vi "AddNewToneParamWave.vi"(1 "Phase  [°]":dbl format="%#_16g", 2 "Phase Selection":u16(ring) items=["Value", "Default", "Minimum", "Maximum"], 4 "Amplitude  [V]":dbl=1.0 format="%#_16g", 5 "Frequency [Hz]":dbl=1000000.0 format="%#_16e", 6 "Amplitude Selection":u16(ring) items=["Value", "Default", "Minimum", "Maximum"], 7 "Frequency Selection":u16(ring) items=["Value", "Default", "Minimum", "Maximum"], 8 "error in (no error)":errorcluster, 10 "ParamWave Name":string, 11 "VISA resource name":refnum<visa-resource-name>) -> (0 "error out":errorcluster, 3 "VISA resource name out":refnum<visa-resource-name>)   [LabVIEW 2020, in "Active Technologies AWG3000.lvlib"]
uses:
  Active Technologies AWG3000.lvlib
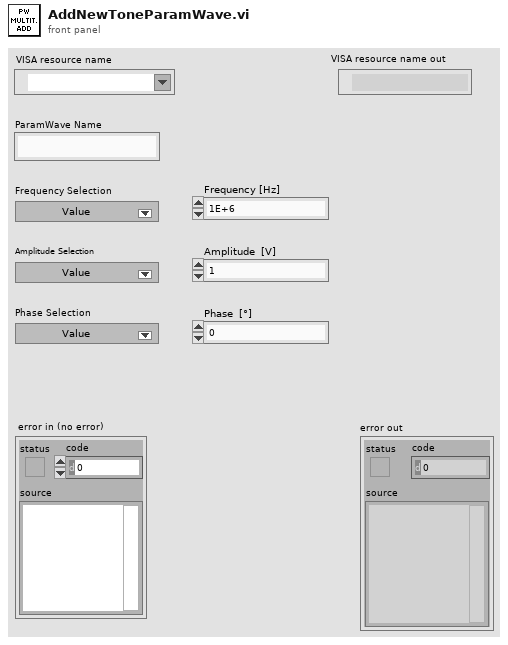
[diagram p1: front panel]
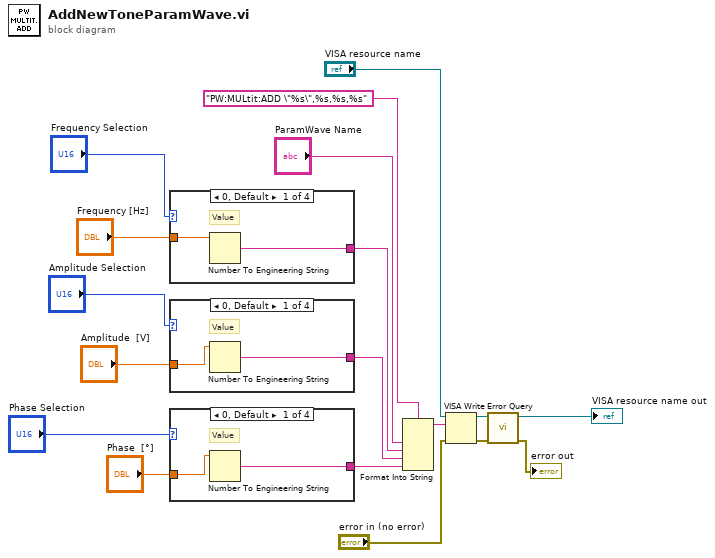
[diagram p0: block diagram]
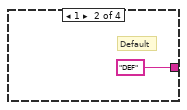
[diagram p2: hidden frame]
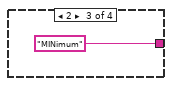
[diagram p3: hidden frame]
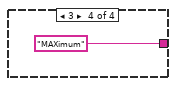
[diagram p4: hidden frame]
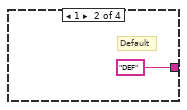
[diagram p5: hidden frame]
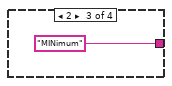
[diagram p6: hidden frame]
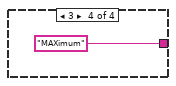
[diagram p7: hidden frame]
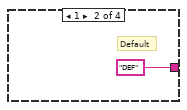
[diagram p8: hidden frame]
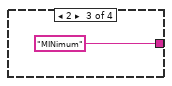
[diagram p9: hidden frame]
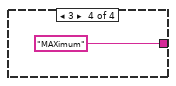
[diagram p10: hidden frame]
diagram:
  n1 = case shown="0, Default" "Frequency Selection" {
    tunnel: [w20 "DEF" ("write buffer") "MINimum" ("write buffer") "MAXimum" ("write buffer")] -> w9
    tunnel: "Frequency [Hz]" -> [w19 _ _ _]
    frame 0, Default {
      # "Value"
      n2 = Number To Engineering String(4:w19) -> (0:w20:string)  [unwired: 3 in]
    }
    frame 1 {
      # "Default"
    }
    frame 2 {
    }
    frame 3 {
    }
  }
  n3 = case shown="0, Default" "Amplitude Selection" {
    tunnel: [w25 "DEF" ("write buffer") "MINimum" ("write buffer") "MAXimum" ("write buffer")] -> w2
    tunnel: "Amplitude  [V]" -> [w24 _ _ _]
    frame 0, Default {
      # "Value"
      n4 = Number To Engineering String(4:w24) -> (0:w25:string)  [unwired: 3 in]
    }
    frame 1 {
      # "Default"
    }
    frame 2 {
    }
    frame 3 {
    }
  }
  n5 = case shown="0, Default" "Phase Selection" {
    tunnel: [w30 "DEF" ("write buffer") "MINimum" ("write buffer") "MAXimum" ("write buffer")] -> w1
    tunnel: "Phase  [°]" -> [w29 _ _ _]
    frame 0, Default {
      # "Value"
      n6 = Number To Engineering String(4:w29) -> (0:w30:string)  [unwired: 3 in]
    }
    frame 1 {
      # "Default"
    }
    frame 2 {
    }
    frame 3 {
    }
  }
  n7 = Format Into String(format string="PW:MULtit:ADD \"%s\",%s,%s,%s" ("write buffer"), "ParamWave Name", w9, w2, w1) -> (resulting string=w8:string)  [unwired: 2 in, 1 out]
  n8 = VISA Write(VISA resource name="VISA resource name", write buffer=w8, error in (no error)="error in (no error)") -> (VISA resource name out=w16:refnum<visa-resource-name>, error out=w15:errorcluster)  [unwired: 1 out]
  n9 = call "Error Query.vi"("error in (no error)"=w15, "VISA resource name"=w16) -> ("error out"=→"error out":errorcluster, "VISA resource name out"=→"VISA resource name out":refnum<visa-resource-name>)  [unwired: 6 in, 2 out]
